vi "macro_Ctrl_HolonomicExecute.vi"() -> ()   [LabVIEW 2019]
uses:
  <vilib>/Rock Robotics/WPI/ThirdParty/JAS_Junk/TrajLib/Trajectory_Library.lvlib
  <vilib>/Rock Robotics/WPI/ThirdParty/JAS_Junk/TrajLib/TypeDef/CHASSIS_SPEEDS.ctl
  <vilib>/Rock Robotics/WPI/ThirdParty/JAS_Junk/TrajLib/TypeDef/ROTATION2D.ctl
  <vilib>/Rock Robotics/WPI/ThirdParty/JAS_Junk/TrajLib/TypeDef/TRANSLATION2D.ctl
  <vilib>/Rock Robotics/WPI/ThirdParty/JAS_Junk/TrajLib/TypeDef/POSE2D.ctl
  TypeDef/PathPlannerPathConstraints.ctl
  TypeDef/PathPlannerTrajectoryState.ctl
panel:
  in  "Reset":bool
  in  "PathPlannerState":T1={"TimeSeconds"=0.0, "VelocityMPS"=0.0, "AccerationMpsSq"=0.0, "HeadingAngularVelRadPerSec"=0.0, "PositionMeters"={"X"=0.0, "Y"=0.0}, "Heading"={"VALUE"=0.0, "COS"=1.0, "SIN"=0.0}, "TargetHolonomicRotation"={"VALUE"=0.0, "COS"=1.0, "SIN"=0.0}, "CurvatureRadPerMeter"=0.0, "PathPlannerConstraints"={"MaxVelocityMps;"=0.0, "MaxAccelerationMpsSq;"=0.0, "MaxAngularVelRadPsEc;"=0.0, "MaxAngularAccRadPSecSq"=0.0, "Exists"=FALSE}, "DeltaPos"=0.0} {"TargetHolonomicRotation"."SIN" format="%13.4f"; "TargetHolonomicRotation"."COS" format="%13.4f"; "TargetHolonomicRotation"."VALUE" format="%13.4f"; "Heading"."SIN" format="%13.4f"; "Heading"."COS" format="%13.4f"; "Heading"."VALUE" format="%13.4f"; "PositionMeters"."Y" format="%14.3f"; "PositionMeters"."X" format="%14.3f"}
  in  "currentPose":T5={"TRANSLATION"={"X"=0.0, "Y"=0.0}, "ROTATION"={"VALUE"=0.0, "COS"=1.0, "SIN"=0.0}} {"ROTATION"."SIN" format="%13.4f"; "ROTATION"."COS" format="%13.4f"; "ROTATION"."VALUE" format="%13.4f"; "TRANSLATION"."Y" format="%14.3f"; "TRANSLATION"."X" format="%14.3f"}
  out "Position Error M":dbl
  out "At Reference":bool
  out "calcChassisSpeed":T6 {"vOmega" format="%10.3f"; "vY" format="%10.3f"; "vX" format="%10.3f"}
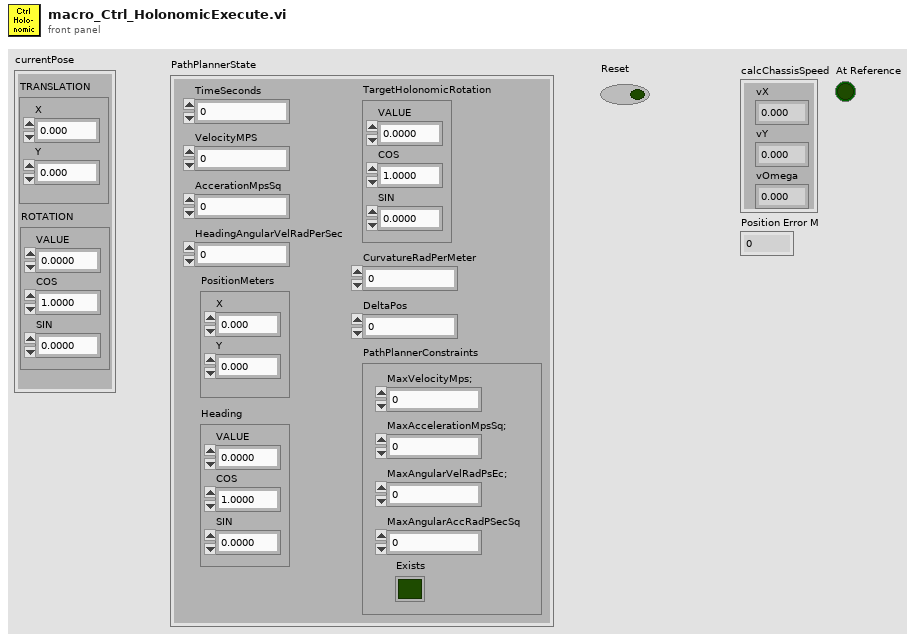
[diagram p1: front panel]
types:
  T1 = typedef "PathPlannerTrajectoryState.ctl" = cluster{"TimeSeconds":dbl, "VelocityMPS":dbl, "AccerationMpsSq":dbl, "HeadingAngularVelRadPerSec":dbl, "PositionMeters":T2, "Heading":T3, "TargetHolonomicRotation":T3, "CurvatureRadPerMeter":dbl, "PathPlannerConstraints":T4, "DeltaPos":dbl}
  T2 = typedef "Trajectory_Library.lvlib/TRANSLATION2D.ctl" = cluster{"X":dbl, "Y":dbl}
  T3 = typedef "Trajectory_Library.lvlib/ROTATION2D.ctl" = cluster{"VALUE":dbl, "COS":dbl, "SIN":dbl}
  T4 = typedef "PathPlannerPathConstraints.ctl" = cluster{"MaxVelocityMps;":dbl, "MaxAccelerationMpsSq;":dbl, "MaxAngularVelRadPsEc;":dbl, "MaxAngularAccRadPSecSq":dbl, "Exists":bool}
  T5 = typedef "Trajectory_Library.lvlib/POSE2D.ctl" = cluster{"TRANSLATION":T2, "ROTATION":T3}
  T6 = typedef "Trajectory_Library.lvlib/CHASSIS_SPEEDS.ctl" = cluster{"vX":dbl, "vY":dbl, "vOmega":dbl}
  T7 = typedef "Trajectory_Library.lvlib/PID_TUNING.ctl" = cluster{"Kp":dbl, "Ki":dbl, "Kd":dbl, "MaximumIntegral":dbl, "MinimumIntegral":dbl}
  T8 = typedef "Trajectory_Library.lvlib/PROFILED_PID_CONTROLLER.ctl" = cluster{"Controller":T9, "Goal":T10, "Setpoint":T10, "Constraint":T11}
  T9 = typedef "Trajectory_Library.lvlib/PID_CONTROLLER.ctl" = cluster{"Kp":dbl, "Ki":dbl, "Kd":dbl, "Period":dbl, "Max_Integral":dbl, "Min_Integral":dbl, "Max_Input":dbl, "Min_Input":dbl, "Continuous":bool, "PositionError":dbl, "VelocityError":dbl, "PrevError":dbl, "TotalError":dbl, "PositionTolerance":dbl, "VelocityTolerance":dbl, "SetPoint":dbl, "Kf":dbl, "Prev_Deriv":dbl, "Prev_Deriv 2":dbl, "DerivativeFilter":bool, "Min_Output":dbl, "Max_Output":dbl, "Prev_F_P":dbl, "Prev_F_P_2":dbl, "AntiWindupActive":bool, "Measurement":dbl}
  T10 = typedef "Trajectory_Library.lvlib/TRAPEZOID_PROFILE_STATE.ctl" = cluster{"Position":dbl, "Velocity":dbl}
  T11 = typedef "Trajectory_Library.lvlib/TRAPEZOID_PROFILE_CONSTRAINT.ctl" = cluster{"MaxVelocity":dbl, "MaxAcceleration":dbl}
  T12 = typedef "PathPlannerCtrlHolConfig.ctl" = cluster{"HOLONOMIC_CTRL_PACK_TUNING":T13, "Max Wheel Speed M/S":dbl, "Tolerance SI":T5, "Drive Base Radius M":dbl}
  T13 = typedef "Trajectory_Library.lvlib/HOLONOMIC_PACK_TUNING.ctl" = cluster{"X PID Tuning":T7, "Y PID Tuning":T7, "thetaProfiledPID_CTRL":T8}
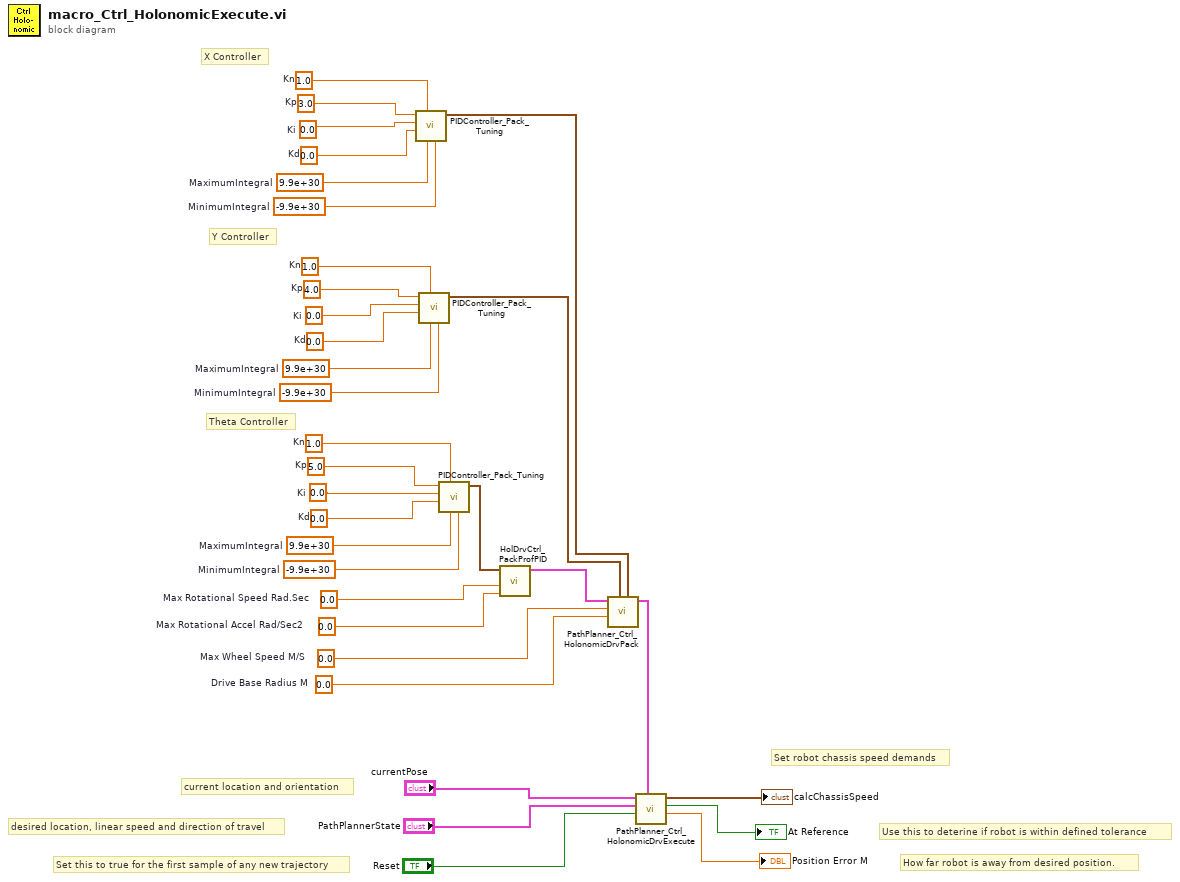
[diagram p0: block diagram]
diagram:
  w2 = 0.0  # Drive Base Radius M
  w3 = 0.0  # Max Wheel Speed M/S
  w15 = 1.0  # Kn
  w18 = 5.0  # Kp
  w27 = 0.0  # Ki
  w28 = 0.0  # Kd
  w29 = 9.9e+30  # MaximumIntegral
  w30 = -9.9e+30  # MinimumIntegral
  w13 = 1.0  # Kn
  w16 = 3.0  # Kp
  w19 = 0.0  # Ki
  w20 = 0.0  # Kd
  w21 = 9.9e+30  # MaximumIntegral
  w22 = -9.9e+30  # MinimumIntegral
  w14 = 1.0  # Kn
  w17 = 4.0  # Kp
  w23 = 0.0  # Ki
  w24 = 0.0  # Kd
  w25 = 9.9e+30  # MaximumIntegral
  w26 = -9.9e+30  # MinimumIntegral
  w12 = 0.0  # Max Rotational Accel Rad/Sec2
  w11 = 0.0  # Max Rotational Speed Rad.Sec
  # "How far robot is away from desired position."
  # "Use this to deterine if robot is within defined tolerance"
  # "Set robot chassis speed demands"
  # "Set this to true for the first sample of any new trajectory"
  # "desired location, linear speed and direction of travel"
  # "current location and orientation"
  # "Theta Controller"
  # "Y Controller"
  # "X Controller"
  n1 = call <vilib>:"PIDController_Pack_Tuning.vi"("MinimumIntegral"=w22, "MaximumIntegral"=w21, "Kn"=w13, "Kd"=w20, "Ki"=w19, "Kp"=w16) -> ("PID Tuning"=w6:T7)  [unwired: 5 in]
  n2 = call <vilib>:"PIDController_Pack_Tuning.vi"("MinimumIntegral"=w26, "MaximumIntegral"=w25, "Kn"=w14, "Kd"=w24, "Ki"=w23, "Kp"=w17) -> ("PID Tuning"=w5:T7)  [unwired: 5 in]
  n3 = call <vilib>:"PIDController_Pack_Tuning.vi"("MinimumIntegral"=w30, "MaximumIntegral"=w29, "Kn"=w15, "Kd"=w28, "Ki"=w27, "Kp"=w18) -> ("PID Tuning"=w10:T7)  [unwired: 5 in]
  n4 = call <vilib>:"HolDrvCtrl_PackProfPID.vi"("Max Accel"=w12, "Max Speed"=w11, "Theta PID Tuning"=w10) -> ("Theta PID CONTROLLER"=w4:T8)  [unwired: 8 in]
  n5 = call "PathPlanner_Ctrl_HolonomicDrvPack.vi"("X PID Tuning"=w6, "Y PID Tuning"=w5, "Drive Base Radius M"=w2, "Max Wheel Speed M/S"=w3, "thetaProfiledPID_CTRL"=w4) -> ("PathPlanner_Ctrl_HolDrvConfig"=w7:T12)  [unwired: 6 in]
  n6 = call "PathPlanner_Ctrl_HolonomicDrvExecute.vi"("PathPlanner_Ctrl_HolDrvConfig"=w7, "Reset"="Reset", "PathPlannerState"="PathPlannerState", "Current Pose SI"="currentPose") -> ("Position Error M"=→"Position Error M":dbl, "At Reference"=→"At Reference":bool, "calcChassisSpeed"=→"calcChassisSpeed":T6)  [unwired: 4 in, 1 out]
